vi "Digital Write 1 Channel.vi"(7 "DAQ Module":i32, 8 "error constant":errorcluster, 9 "Value":bool=TRUE, 10 "Channel":i32, 11 "NI-DAQ.lvclass":refnum<class "NI-DAQ.lvclass">) -> (0 "error IO":errorcluster, 3 "NI-DAQ.lvclass 2":refnum<class "NI-DAQ.lvclass">)   [LabVIEW 2016, in "NI-DAQ.lvclass"]
uses:
  NI-DAQ.lvclass
  NI-DAQ.lvclass/NI-DAQ.ctl
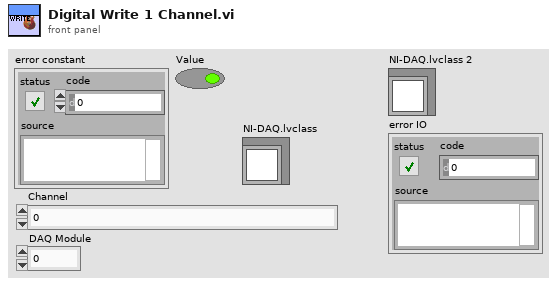
[diagram p1: front panel]
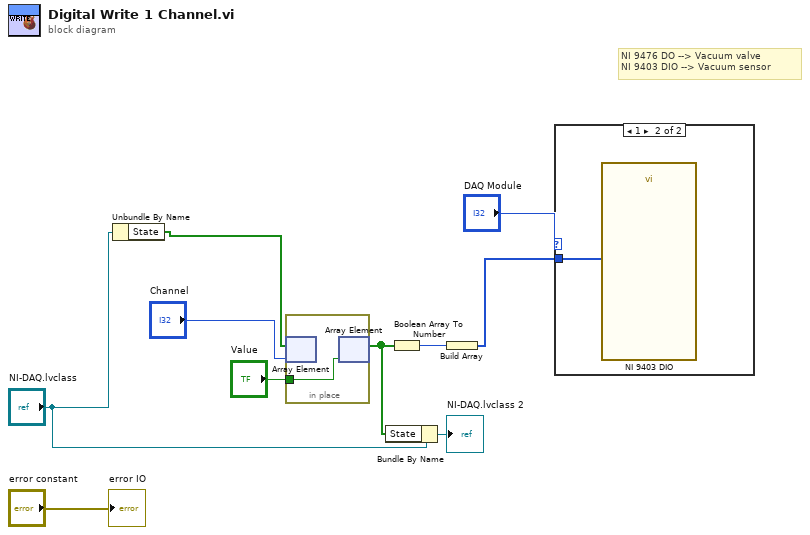
[diagram p0: block diagram]
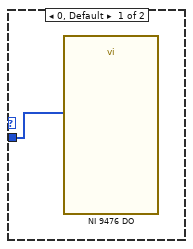
[diagram p2: hidden frame]
diagram:
  # "NI 9476 DO --> Vacuum valve\nNI 9403 DIO --> Vacuum sensor"
  n1 = Unbundle By Name("NI-DAQ.lvclass") -> ("State"=w2:bool[])
  n2 = in-place {
    in-place-border: "Value" -> [w11]
    n3 = in-place-array #1(w2, "Channel") -> ()  [unwired: 1 out]
    n4 = in-place-array #1(w11) -> (w3:bool[])  [unwired: 1 out]
  }
  n5 = Bundle By Name(cluster="NI-DAQ.lvclass", "State"=w3) -> (→"NI-DAQ.lvclass 2":refnum<class "NI-DAQ.lvclass">)
  n6 = Boolean Array To Number(Boolean array=w3) -> (number=w4:u32)
  n7 = Build Array(w4) -> (w6:u32[])
  n8 = case shown="1" "DAQ Module" {
    tunnel: w6 -> [w12 w13]
    frame 0, Default {
      n9 = call "NI 9476 DO"("data"=w12) -> ()  [unwired: 17 in, 2 out]
    }
    frame 1 {
      n10 = call "NI 9403 DIO"("data"=w13) -> ()  [unwired: 17 in, 2 out]
    }
  }
  "error IO" <- "error constant"
